vi "G#Object_StartExternalCreateProcess.vi"(5 "error in (no error)":errorcluster) -> (19 "error out":errorcluster)   [LabVIEW 2017, in "G#Object.lvclass"]
doc: "Starts an external create process in the background. This process will create and own all G# objects and prevent LabVIEW garbage collector to clear them. It is stopped when running the garbage collector. This is useful if having multiple top-level applications, but is not needed with a single top-level application."
uses:
  G#Object.lvclass
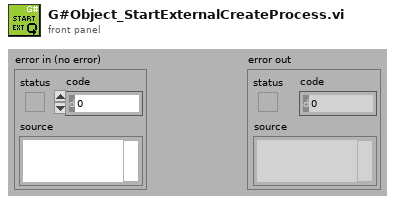
[diagram p1: front panel]
types:
  T1 = enum16{"Initialize", "Register", "Unregister", "Clear"}
  T2 = enum32{"Bad", "Idle", "Run top level", "Running"}
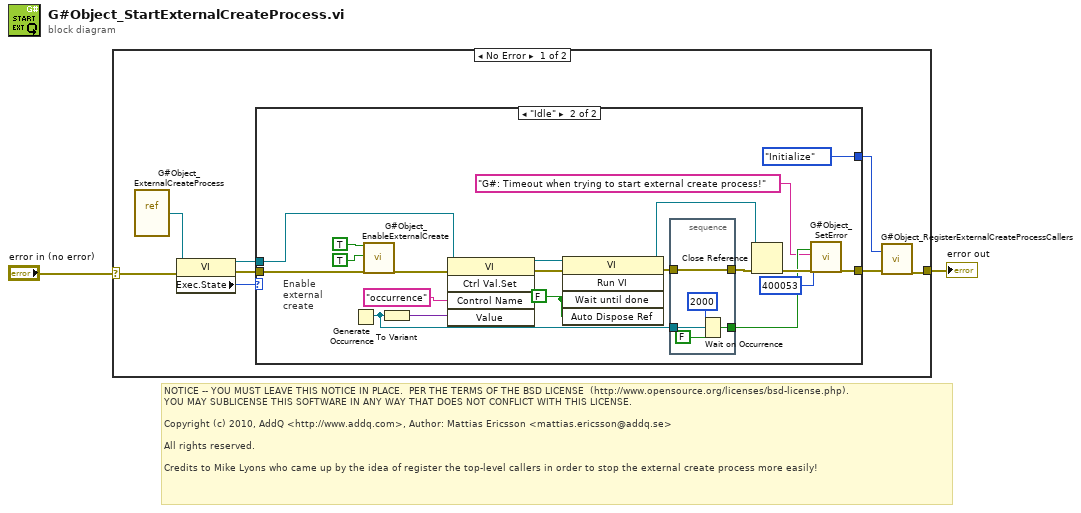
[diagram p0: block diagram]
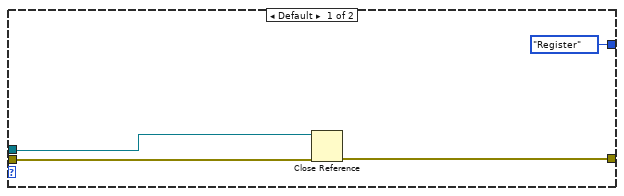
[diagram p2: hidden frame]
diagram:
  # "NOTICE -- YOU MUST LEAVE THIS NOTICE IN PLACE.  PER THE TERMS OF THE BSD LICENSE  (http://www.opensource.org/licenses/bsd-license.php).\nYOU MAY SUBLICENSE THIS SOFTWARE IN ANY WAY THAT DOES NOT CONFLICT WITH THIS LICENSE.\n\nCopyright (c) 2010, AddQ <http://www.addq.com>, Author: Mattias Ericsson <mattias.ericsson@addq.se>\n\nAll rights reserved.\n\nCredits to Mike Lyons who came up by the idea of register the top-level callers in order to stop the external create process more easily!"
  n1 = case shown="No Error" "error in (no error)" {
    selector: "error in (no error)" -> [w6 w40]
    tunnel: [w4 w40] -> w1
    frame No Error {
      n2 = vi-ref "G#Object_ExternalCreateProcess.vi"() -> (w10:refnum<vi>)
      n3 = property class="VI"(reference=w10, error in=w6) -> (reference out=w7:refnum<vi>, error out=w8:errorcluster, "Exec.State"=w9:T2)
      n4 = case shown="\"Idle\"" w9 {
        tunnel: w8 -> [w14 w18]
        tunnel: w7 -> [w12 w34]
        tunnel: [w13 w16] -> w5
        tunnel: [T1."Register" ("Action") T1."Initialize" ("Action")] -> w3
        frame Default {
          n5 = Close Reference(reference=w12, error in (no error)=w14) -> (error out=w13:errorcluster)
        }
        frame "Idle" {
          w29 = FALSE ("Wait Until Done")
          # "Enable\nexternal\ncreate"
          n6 = Generate Occurrence() -> (w27:refnum<k4>)
          n7 = call "G#Object_EnableExternalCreate.vi"("set (F)"=TRUE ("set"), "external create enable (F)"=TRUE ("external create enable"), "error in (no error)"=w18) -> ("error out"=w19:errorcluster)  [unwired: 14 in, 2 out]
          n8 = To Variant(anything=w27) -> (Variant=w32:variant)
          n9 = invoke class="VI" method="Ctrl Val.Set"(reference=w34, error in=w19, "Control Name"="occurrence", "Value"=w32) -> (reference out=w30:refnum<vi>, error out=w31:errorcluster)  [unwired: 1 in, 3 out]
          n10 = invoke class="VI" method="Run VI"(reference=w30, error in=w31, "Wait until done"=w29, "Auto Dispose Ref"=w29) -> (reference out=w25:refnum<vi>, error out=w28:errorcluster)  [unwired: 1 in, 3 out]
          n11 = stacked-sequence {
            tunnel: w28 -> [w37]
            tunnel: w27 -> [w39]
            tunnel: [w37] -> w26
            tunnel: [w36] -> w23
            frame #0 {
              n12 = Wait on Occurrence(1:FALSE ("ignore previous (T)"), 2:w39, 3:2000 ("ms timeout (-1)")) -> (0:w36:bool)
            }
          }
          n13 = Close Reference(reference=w25, error in (no error)=w26) -> (error out=w24:errorcluster)
          n14 = call "G#Object_SetError.vi"("error (F)"=w23, "source"="G#: Timeout when trying to start external create process!", "code"=400053, "error in (no error)"=w24) -> ("error out"=w16:errorcluster)  [unwired: 15 in]
        }
      }
      n15 = call "G#Object_RegisterExternalCreateProcessCallers.vi"("Action"=w3, "error in (no error)"=w5) -> ("error out"=w4:errorcluster)  [unwired: 16 in, 1 out]
    }
    frame Error {
    }
  }
  "error out" <- w1
